vi "Camera_AutoGain.vi"(2 "SRV In":string) -> (1 "Gain set":u8, 4 "SRV Out":string="169.254.0.10")   [LabVIEW 2009]
panel:
  in  "Gain":u16(ring) items=["AGC enable"=4, "AWB enable"=2, "AEC enable"=1, "All on"=7, "All off"=0]
  out "data out":string
  # "This LabVIEW item is deprecated.\n\nIt is believed to be unused and will be removed in a future version of SRV."
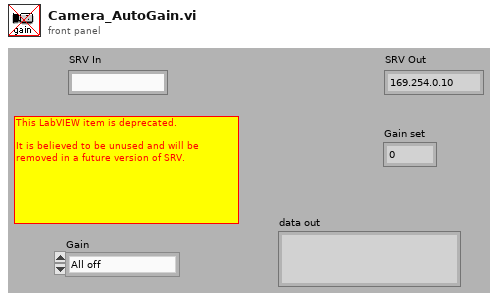
[diagram p1: front panel]
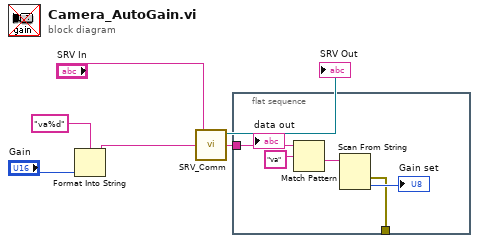
[diagram p0: block diagram]
diagram:
  n1 = Format Into String(format string="va%d", "Gain") -> (resulting string=w1:string)  [unwired: 2 in, 1 out]
  n2 = call "SRV_Comm.vi"("Command Sent"=w1, "SRV In"="SRV In") -> ("Reply"=w6:string, "SRV Out"=→"SRV Out":refnum<k5>)  [unwired: 1 in, 1 out]
  n3 = flat-sequence {
    tunnel: w6 -> [w11]
    tunnel: [w7] -> _
    frame #0 {
      n4 = Match Pattern(string=w11, regular expression="va" ("Command Sent")) -> (after substring=w9:string)  [unwired: 1 in, 3 out]
      n5 = Scan From String(input string=w9) -> (error out=w7:errorcluster, output 1=→"Gain set":u8)  [unwired: 4 in, 2 out]
      "data out" <- w11
    }
  }
